vi "Translator.FormatMessage.vi"(8 "error in (no error)":errorcluster, 9 "Arguments":variant[](array[variant]), 10 "Msg":string) -> (0 "error out":errorcluster, 2 "Translated Msg":string)   [LabVIEW 2016]
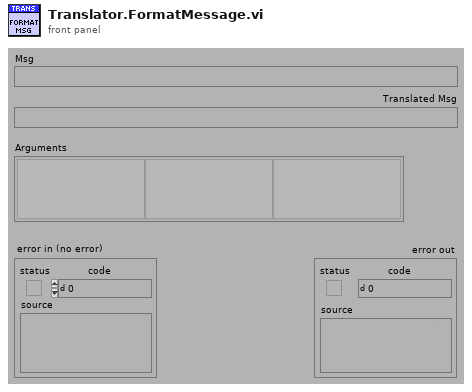
[diagram p1: front panel]
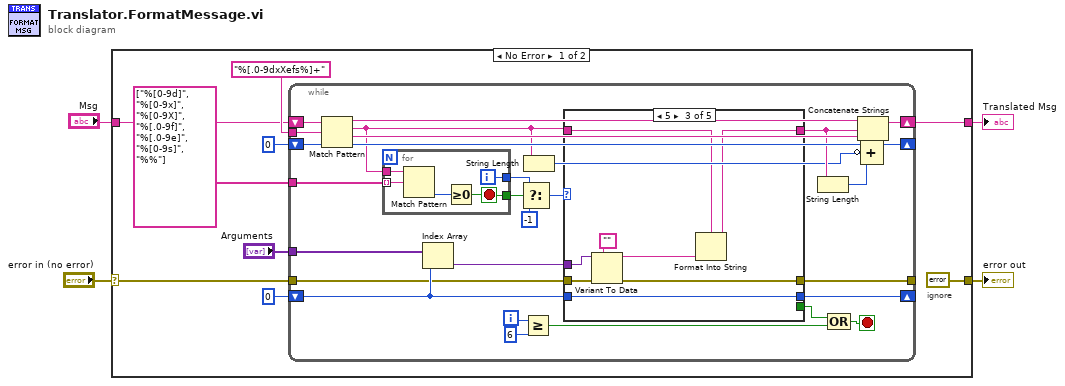
[diagram p0: block diagram]
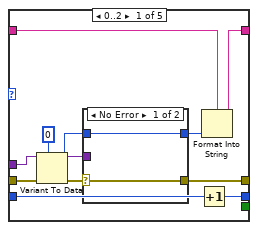
[diagram p2: hidden frame]
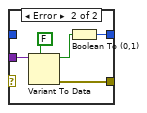
[diagram p3: hidden frame]
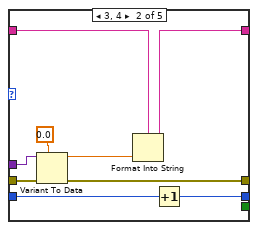
[diagram p4: hidden frame]
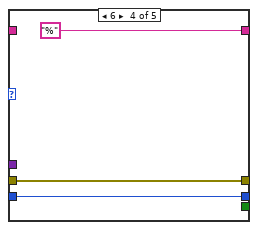
[diagram p5: hidden frame]
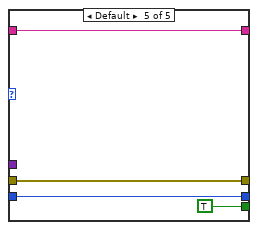
[diagram p6: hidden frame]
diagram:
  n1 = case shown="No Error" "error in (no error)" {
    selector: "error in (no error)" -> [w6 w91]
    tunnel: [w12 w90] -> w4
    tunnel: [errorcluster {"status"=FALSE, "code"=0, "source"=""} ("error out") w91] -> w3
    tunnel: "Msg" -> [w5 w90]
    frame No Error {
      # "ignore"
      n2 = while {
        tunnel: string[] ["%[0-9d]", "%[0-9x]", "%[0-9X]", "%[.0-9f]", "%[.0-9e]", "%[0-9s]", "%%"] -> [w37]
        shift-right: [w41] -> _
        shift-left: 0 -> [w39]
        shift-right: [w18] -> _
        shift-left: 0 -> [w33]
        tunnel: "Arguments" -> [w40]
        shift-right: [w25] -> w12
        shift-left: w5 -> [w35]
        tunnel: "%[.0-9dxXefs%]+" -> [w34]
        tunnel: w6 -> [w36]
        tunnel: [w23] -> _
        i -> [w17]
        stop <- w24 stop-if-true
        n3 = Match Pattern(string=w35, regular expression=w34, offset (0)=w33) -> (before substring=w27:string, match substring=w22:string, after substring=w26:string, offset past match=w32:i32)
        n4 = for {
          tunnel: w22 -> [w89]
          tunnel: w37 -> [w88] mode=indexing
          tunnel: [w85] -> w29
          tunnel: [w86] -> w31
          i -> [w85]
          stop <- w86 stop-if-true
          n5 = Match Pattern(string=w89, regular expression=w88) -> (offset past match=w87:i32)  [unwired: 1 in, 3 out]
          n6 = Greater Or Equal To 0?(x=w87) -> (x >= 0?=w86:bool)
        }
        n7 = Index Array(array=w40, index=w39) -> (element=w38:variant)
        n8 = Select(t=w29, s=w31, f=-1) -> (s? t:f=w30:i32)
        n9 = Greater Or Equal?(x=w17, y=6) -> (x >= y?=w15:bool)
        n10 = String Length(string=w22) -> (length=w20:i32)
        n11 = case shown="5" w30 {
          tunnel: w39 -> [w49 w65 w76 w78 w84]
          tunnel: [w52 w68 w77 w78 w84] -> w41
          tunnel: w22 -> [w51 w67 w71 _ w81]
          tunnel: w38 -> [w43 w63 w73 _ _]
          tunnel: [w47 w61 w69 "%" ("Msg") w81] -> w21
          tunnel: [_ _ _ _ TRUE] -> w14
          tunnel: w36 -> [w48 w62 w74 w79 w82]
          tunnel: [w42 w60 w70 w79 w82] -> w23
          frame 0..2 {
            n12 = Variant To Data(error in=w48, type=i64 0, Variant=w43) -> (data=w45:i64, error out=w46:errorcluster)
            n13 = case shown="No Error" w46 {
              selector: w46 -> [w54 _]
              tunnel: [w54 w57] -> w42
              tunnel: [w53 w55] -> w44
              tunnel: w45 -> [w53 _]
              tunnel: w43 -> [_ w58]
              frame No Error {
              }
              frame Error {
                n14 = Variant To Data(type=FALSE, Variant=w58) -> (data=w56:bool, error out=w57:errorcluster)  [unwired: 1 in]
                n15 = Boolean To (0,1)(Boolean=w56) -> (0, 1=w55:i16)
              }
            }
            n16 = Increment(x=w49) -> (x+1=w52:i32)
            n17 = Format Into String(format string=w51, w44) -> (resulting string=w47:string)  [unwired: 2 in, 1 out]
          }
          frame 3, 4 {
            n18 = Variant To Data(error in=w62, type=0.0, Variant=w63) -> (data=w64:dbl, error out=w60:errorcluster)
            n19 = Format Into String(format string=w67, w64) -> (resulting string=w61:string)  [unwired: 2 in, 1 out]
            n20 = Increment(x=w65) -> (x+1=w68:i32)
          }
          frame 5 {
            n21 = Variant To Data(error in=w74, type="", Variant=w73) -> (data=w72:string, error out=w70:errorcluster)
            n22 = Format Into String(format string=w71, w72) -> (resulting string=w69:string)  [unwired: 2 in, 1 out]
            n23 = Increment(x=w76) -> (x+1=w77:i32)
          }
          frame 6 {
          }
          frame Default {
          }
        }
        n24 = String Length(string=w21) -> (length=w19:i32)
        n25 = Compound Arithmetic op=OR(w14, w15) -> (w24:bool)
        n26 = Concatenate Strings(w27, w21, w26) -> (w25:string)
        n27 = Compound Arithmetic op=ADD(w32, invert w20, w19) -> (w18:i32)
      }
    }
    frame Error {
    }
  }
  "Translated Msg" <- w4
  "error out" <- w3
